vi "Initialize UUIDs.vi"(8 "error in (no error)":errorcluster, 11 "CubeLogger in":refnum<class "CubeLogger.lvclass">) -> (0 "error out":errorcluster, 2 "UUID[]":string[](array[string]), 3 "CubeLogger out":refnum<class "CubeLogger.lvclass">)   [LabVIEW 2018, in "CubeLogger.lvclass"]
uses:
  CubeLogger.lvclass
  CubeLogger.lvclass/CubeLogger.ctl
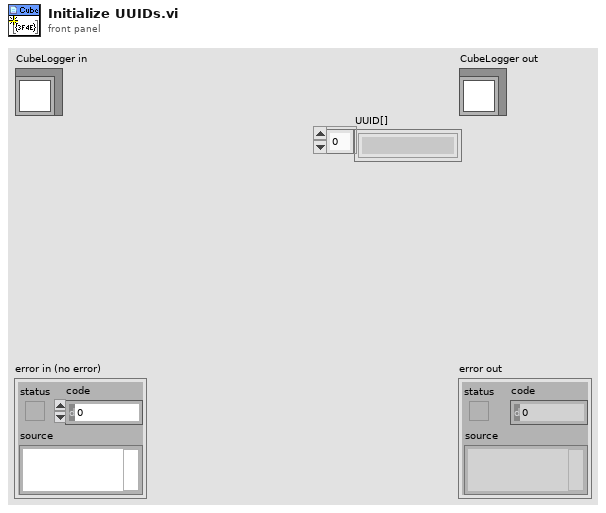
[diagram p1: front panel]
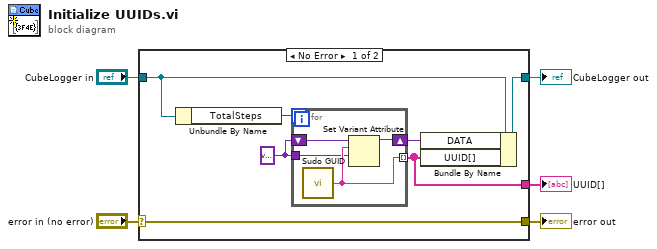
[diagram p0: block diagram]
diagram:
  n1 = case shown="No Error" "error in (no error)" {
    selector: "error in (no error)" -> [w12 w18]
    tunnel: [w12 w18] -> w4
    tunnel: [w7 w17] -> w2
    tunnel: "CubeLogger in" -> [w11 w17]
    tunnel: [w6 _] -> w1
    frame No Error {
      w8 = variant
      n2 = Unbundle By Name(w11) -> ("TotalSteps"=w10:i32)
      n3 = for {
        N: w10 -> [_]
        shift-right: [w15] -> w9
        shift-left: w8 -> [w16]
        tunnel: [w14] -> w6 mode=indexing
        tunnel: w8 -> [w13]
        n4 = call "Sudo GUID.vi"() -> ("GUID String"=w14:string)  [unwired: 5 in]
        n5 = Set Variant Attribute(Variant=w16, name=w14, value=w13) -> (Variant out=w15:variant)  [unwired: 1 in, 2 out]
      }
      n6 = Bundle By Name(cluster=w11, "DATA"=w9, "UUID[]"=w6) -> (w7:refnum<class "CubeLogger.lvclass">)
    }
    frame Error {
    }
  }
  "error out" <- w4
  "CubeLogger out" <- w2
  "UUID[]" <- w1
